vi "Simple Solenoid.vi"() -> ()   [LabVIEW 2018]
doc: "Simple Solenoid Example\n\nThis example shows how to set the value of a Solenoid Channel.\n\nIt works with the PCM (Pneumatic Control Module) communicating with the roboRIO over CAN bus. The PCM must also be supplied with 12V DC from the PDP (Power Distribution Panel).\n\nThe Compressor, Pressure Switch, and Solenoid are all wired to the PCM \n\nThis example expects a USB cable connected from your development PC to the Type B USB Jack (next to the power input) on the roboRIO.\n\nThis example expects the Driver Station to be running."
uses:
  <vilib>/Rock Robotics/WPI/Solenoid/WPI_SolenoidValue.ctl
  <vilib>/Rock Robotics/WPI/Solenoid/WPI_SolenoidSetEnum.vi
  <vilib>/Rock Robotics/WPI/Solenoid/WPI_SolenoidOpenSingle.vi
  <vilib>/Rock Robotics/WPI/Solenoid/WPI_SolenoidChannel.ctl
panel:
  in  "Value to Write 2":bool
  in  "stop 2":bool
  in  "Solenoid Channel":T1
  in  "Value to Write":bool
  in  "stop":bool
  # "Set this input before running."
  # "This can be set while running."
  # "On"
  # "Off"
  # "Wiring Diagram"
  # "Pneumatic Control Module"
  # "To Solenoid"
  # "CAN"
  # "COMPRESSOR OUT"
  # "PRESSURE"
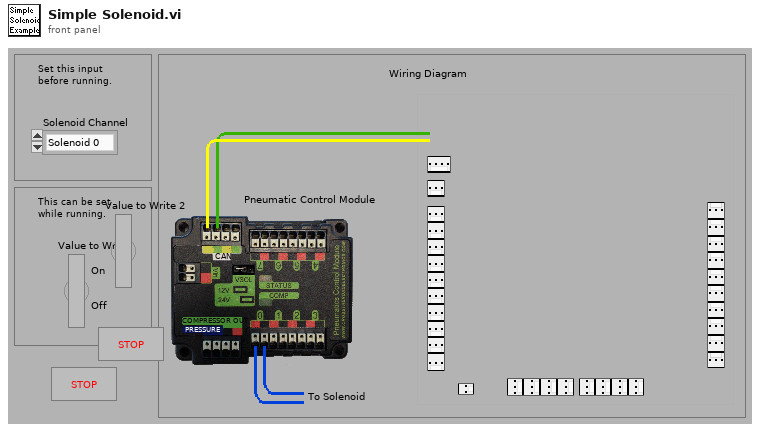
[diagram p1: front panel]
types:
  T1 = typedef "WPI_SolenoidChannel.ctl" = enum8{"Solenoid 0", "Solenoid 1", "Solenoid 2", "Solenoid 3", "Solenoid 4", "Solenoid 5", "Solenoid 6", "Solenoid 7", "Invalid"}
  T2 = typedef "WPI_SolenoidDevRef.ctl" = cluster{"DevStatus":errorcluster, "Pneumatics Control Module":u8, "Forward Solenoid Channel":T1, "Reverse Solenoid Channel":T1}
  T3 = typedef "WPI_SolenoidValue.ctl" = enum16{"Off", "On", "Forward", "Reverse"}
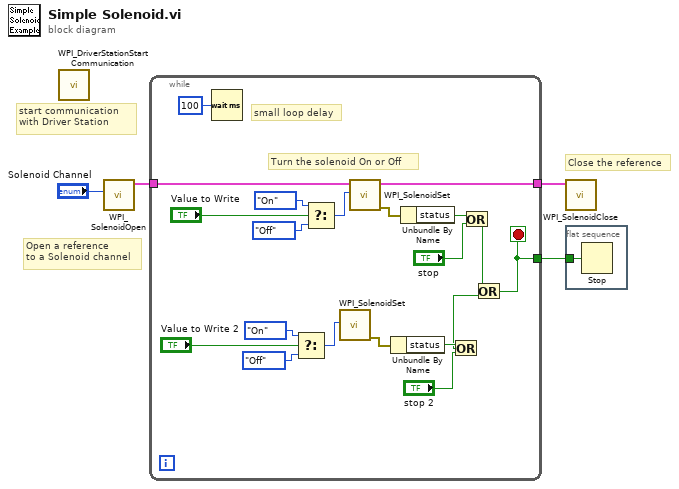
[diagram p0: block diagram]
diagram:
  # "start communication with Driver Station"
  # "Close the reference"
  # "Open a reference \nto a Solenoid channel"
  n1 = call <vilib>:"WPI_DriverStationStart Communication.vi"() -> ()  [unwired: 2 in, 10 out]
  n2 = call-poly <vilib>:"WPI_SolenoidOpen.vi"("Solenoid Channel"="Solenoid Channel") -> ("SolenoidDevRef"=w4:T2)  [unwired: 2 in, 8 out]
  n3 = while {
    tunnel: w4 -> [w23]
    tunnel: [w22] -> w3
    tunnel: [w5] -> w1
    stop <- w5 stop-if-true
    # "small loop delay"
    # "Turn the solenoid On or Off"
    n4 = Wait (ms)(milliseconds to wait=u32 100) -> ()  [unwired: 1 out]
    n5 = Select(t=WPI_SolenoidValue."On" ("Value"), s="Value to Write 2", f=WPI_SolenoidValue."Off" ("Value")) -> (s? t:f=w8:T3)
    n6 = Select(t=WPI_SolenoidValue."On" ("Value"), s="Value to Write", f=WPI_SolenoidValue."Off" ("Value")) -> (s? t:f=w15:T3)
    n7 = call-poly <vilib>:"WPI_SolenoidSet.vi"("Value"=w8) -> ("error out"=w14:errorcluster)  [unwired: 2 in, 8 out]
    n8 = call-poly <vilib>:"WPI_SolenoidSet.vi"("Value"=w15, "SolenoidDevRef"=w23) -> ("error out"=w21:errorcluster, "SolenoidDevRef"=w22:T2)  [unwired: 1 in, 7 out]
    n9 = Unbundle By Name(w14) -> ("status"=w13:bool)
    n10 = Unbundle By Name(w21) -> ("status"=w20:bool)
    n11 = Or(x=w13, y="stop 2") -> (x .or. y?=w7:bool)
    n12 = Or(x=w20, y="stop") -> (x .or. y?=w6:bool)
    n13 = Or(x=w6, y=w7) -> (x .or. y?=w5:bool)
  }
  n14 = call <vilib>:"WPI_SolenoidClose.vi"("SolenoidDevRef"=w3) -> ()  [unwired: 1 in, 10 out]
  n15 = flat-sequence {
    tunnel: w1 -> [w25]
    frame #0 {
      n16 = Stop(stop? (T)=w25) -> ()
    }
  }
